vi "GateSetState.vi"(10 "GateCylState":T1) -> ()   [LabVIEW 2014, in "GateLib.lvlib"]
uses:
  GateLib.lvlib
  <vilib>/Rock Robotics/WPI/Solenoid/WPI_SolenoidValue.ctl
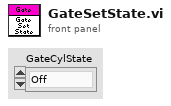
[diagram p1: front panel]
types:
  T1 = typedef "WPI_SolenoidValue.ctl" = enum16{"Off", "On", "Forward", "Reverse"}
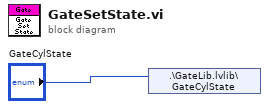
[diagram p0: block diagram]
diagram:
  n1 = shared-variable ".\\GateLib.lvlib\\GateCylState"("GateCylState") -> ()  [unwired: 1 in, 1 out]
